vi "oaa_Get Relative SpeedProfile.vi"(8 "error in (no error)":errorcluster, 11 "speed profile":waveform(dbl)={"t0"=timestamp(0 s since 1904-01-01), "dt"=0.0, "Y"=[]}) -> (0 "error out":errorcluster, 3 "speed profile out":T1 {"speed [RPM]" format="%.2f"; "time [s]" format="%.2f"})   [LabVIEW 2017]
uses:
  <vilib>/addons/Sound and Vibration/Order Analysis/Tach Process/SubVIs/speed profile.ctl
  <vilib>/addons/Sound and Vibration/Order Analysis/Tach Process/SoundVib_TachProcess.lvlib
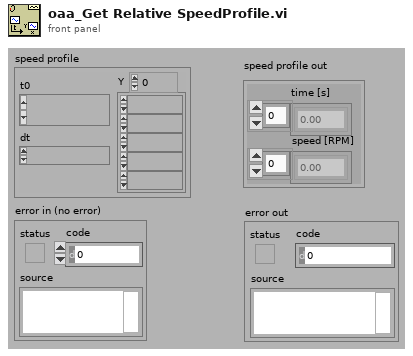
[diagram p1: front panel]
types:
  T1 = typedef "SoundVib_TachProcess.lvlib/speed profile.ctl" = cluster{"time [s]":dbl[], "speed [RPM]":dbl[]}
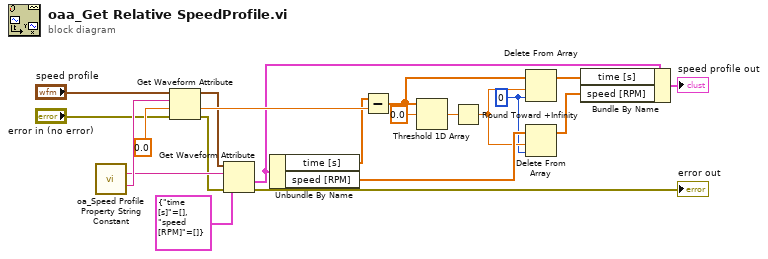
[diagram p0: block diagram]
diagram:
  w8 = 0 ("index")
  n1 = call <vilib>:"oa_Speed Profile Property String Constant.vi"() -> ("speed profile"=w5:string, "elapsed time"=w20:string)  [unwired: 12 in, 2 out]
  n2 = Get Waveform Attribute(4:"error in (no error)", 5:0.0 ("bandwidth [order]"), 6:w20, 7:"speed profile") -> (0:w2:errorcluster, 1:w17:dbl, 3:w3:waveform(dbl))  [unwired: 1 out]
  n3 = Get Waveform Attribute(4:w2, 5:T1 {"time [s]"=[], "speed [RPM]"=[]} ("speed profile"), 6:w5, 7:w3) -> (0:→"error out":errorcluster, 1:w4:T1)  [unwired: 2 out]
  n4 = Unbundle By Name(w4) -> ("time [s]"=w14:dbl[], "speed [RPM]"=w13:dbl[])
  n5 = Subtract(x=w14, y=w17) -> (x-y=w9:dbl[])
  n6 = Threshold 1D Array(2:0.0 ("threshold y"), 3:w9) -> (0:w15:dbl)  [unwired: 1 in]
  n7 = Round Toward +Infinity(x=w15) -> (ceil(x): smallest int >= x=w12:dbl)
  n8 = Delete From Array(array=w9, length=w12, index=w8) -> (array with subset deleted=w10:dbl[])  [unwired: 1 out]
  n9 = Delete From Array(array=w13, length=w12, index=w8) -> (array with subset deleted=w11:dbl[])  [unwired: 1 out]
  n10 = Bundle By Name(cluster=w4, "time [s]"=w10, "speed [RPM]"=w11) -> (→"speed profile out":T1)
